vi "Read Decimal.vi"(11 "MsgSerializer":refnum<class "MsgSerializer.lvclass">) -> (2 "Decimal":T1, 3 "MsgSerializer":refnum<class "MsgSerializer.lvclass">)   [LabVIEW 2020, in "Caraya.lvlib" / "MsgSerializer.lvclass"]
uses:
  MsgSerializer/MsgSerializer.lvclass
  decimal-notation -- enum.ctl
  MsgSerializer/MsgSerializer.lvclass/MsgSerializer.ctl
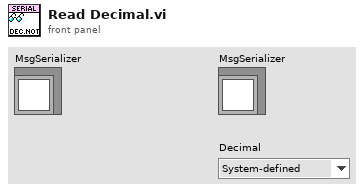
[diagram p1: front panel]
types:
  T1 = typedef "Caraya.lvlib/MsgSerializer.lvclass/decimal-notation -- enum.ctl" = enum16{"System-defined", "dot-notation", "comma-notation"}
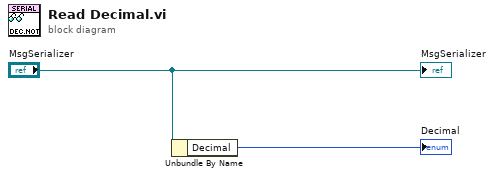
[diagram p0: block diagram]
diagram:
  n1 = Unbundle By Name("MsgSerializer") -> ("Decimal"=→"Decimal":T1)
  "MsgSerializer" <- "MsgSerializer"
